vi "Inlining String.vi"(9 "ExecInlineIfPossible":bool, 11 "ExecInlining":bool) -> (3 "Inline Text":string)   [LabVIEW 2023, in "VIDoc Printer.lvlib" / "VIDoc Printer.lvclass"]
doc: "Converts the Inline information into a printable String."
uses:
  VIDoc Printer.lvclass
  VIDoc Printer.lvclass/VIDoc Printer.ctl
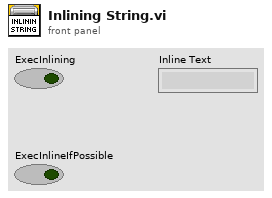
[diagram p1: front panel]
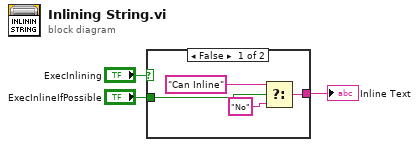
[diagram p0: block diagram]
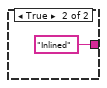
[diagram p2: hidden frame]
diagram:
  n1 = case shown="False" "ExecInlining" {
    tunnel: [w5 "Inlined"] -> w2
    tunnel: "ExecInlineIfPossible" -> [w6 _]
    frame False {
      n2 = Select(t="Can Inline", s=w6, f="No") -> (s? t:f=w5:string)
    }
    frame True {
    }
  }
  "Inline Text" <- w2
